vi "Update Table Data.vi"(8 "error in (no error)":errorcluster, 9 "Stream Names":string[](array[string]), 10 "Data":waveform(dbl)[](array[waveform]), 11 "Plugin in":refnum<class "Historical Table.lvclass">) -> (0 "error out":errorcluster, 3 "Plugin out":refnum<class "Historical Table.lvclass">)   [LabVIEW 2024, in "Historical Table.lvlib" / "Historical Table.lvclass"]
uses:
  Historical Table.lvclass
  Historical Table.lvclass/Historical Table.ctl
  <vilib>/FlexLogger/SDK/PluginSDK.lvlibp
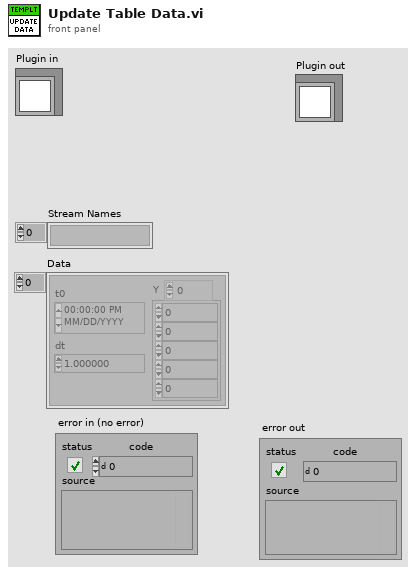
[diagram p1: front panel]
types:
  T1 = enum32{"Invalid", "Standard", "Closed", "Hidden", "Minimized", "Maximized"}
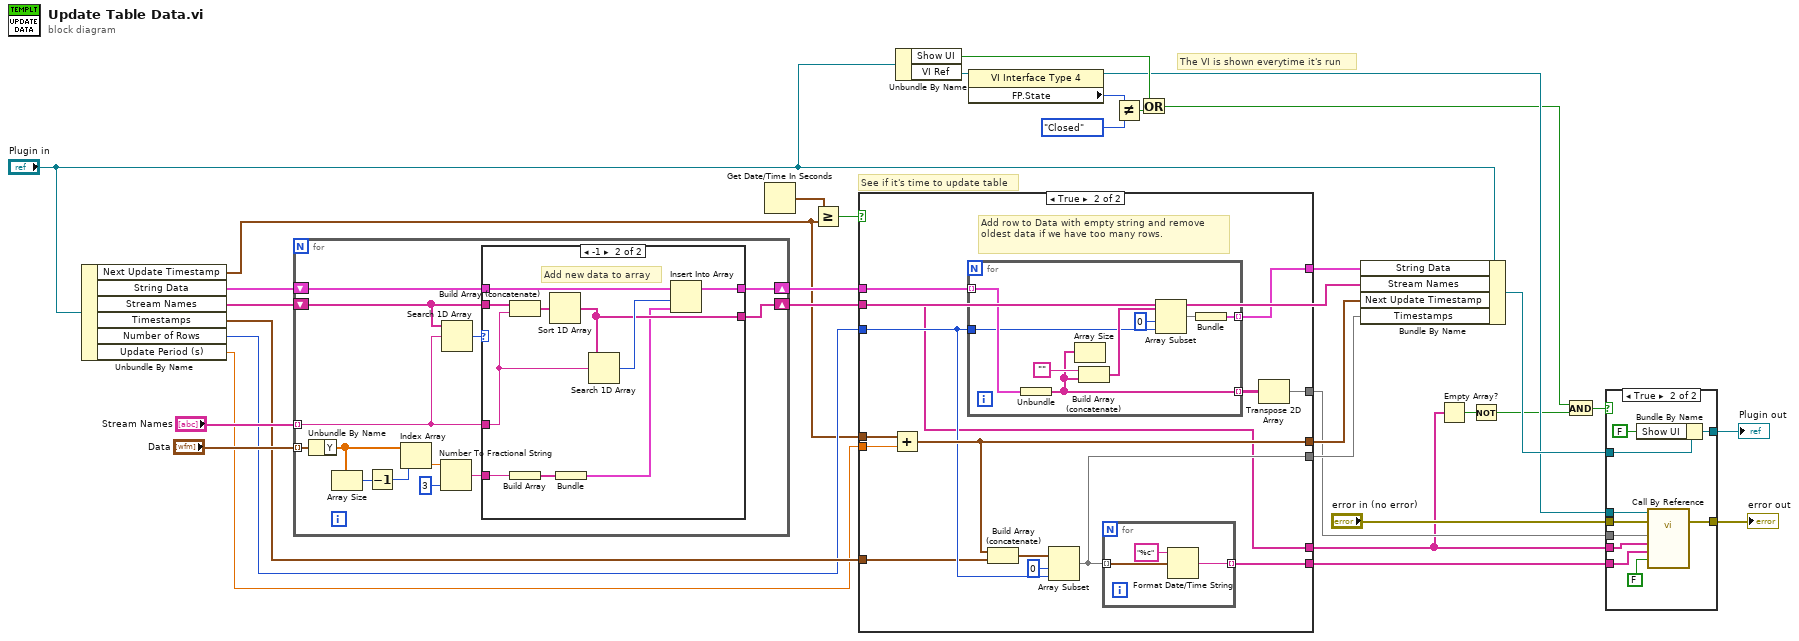
[diagram p0: block diagram]
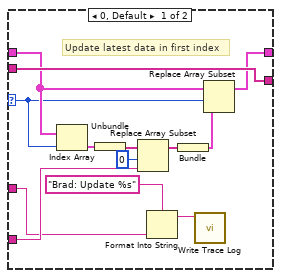
[diagram p3: hidden frame]
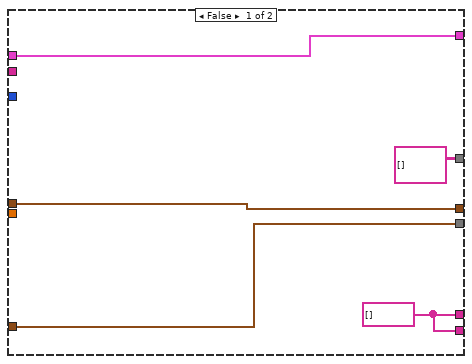
[diagram p4: hidden frame]
diagram:
  # "The VI is shown everytime it's run"
  # "See if it's time to update table"
  n1 = Unbundle By Name("Plugin in") -> ("Next Update Timestamp"=w4:timestamp, "String Data"=w31:cluster{"Data":string[]}[], "Stream Names"=w30:string[], "Timestamps"=w28:timestamp[], "Number of Rows"=w26:i32, "Update Period (s)"=w25:dbl)
  n2 = for {
    tunnel: "Data" -> [w41] mode=indexing
    tunnel: "Stream Names" -> [w45] mode=indexing
    shift-right: [w35] -> w29
    shift-left: w31 -> [w37]
    shift-right: [w34] -> w24
    shift-left: w30 -> [w36]
    n3 = Unbundle By Name(w41) -> ("Y"=w39:dbl[])
    n4 = Array Size(array=w39) -> (size(s)=w38:i32)
    n5 = Decrement(x=w38) -> (x-1=w43:i32)
    n6 = Index Array(array=w39, index=w43) -> (element=w44:dbl)
    n7 = Number To Fractional String(number=w44, precision (6)=i16 3) -> (F-format string=w40:string)  [unwired: 2 in]
    n8 = Search 1D Array(1D array=w36, element=w45) -> (index of element=w46:i32)  [unwired: 1 in]
    n9 = case shown="-1" w46 {
      selector: w46 -> [w56 _]
      tunnel: w36 -> [w59 w69]
      tunnel: w45 -> [w47 w60]
      tunnel: w37 -> [w57 w67]
      tunnel: [w59 w65] -> w34
      tunnel: [w58 w64] -> w35
      tunnel: w40 -> [w53 w63]
      frame 0, Default {
        # "Update latest data in first index"
        n10 = Index Array(array=w57, index=w56) -> (element=w55:cluster{"Data":string[]})
        n11 = Unbundle(w55) -> ("Data"=w54:string[])
        n12 = Replace Array Subset(array=w54, new element=w53, index=0) -> (w51:string[])
        n13 = Format Into String(format string="Brad: Update %s", w47) -> (resulting string=w49:string)  [unwired: 2 in, 1 out]
        n14 = Bundle("Data"=w51) -> (w50:cluster{"Data":string[]})  [unwired: 1 in]
        n15 = call <vilib>:"Write Trace Log.vi"("Message"=w49) -> ()  [unwired: 10 in, 1 out]
        n16 = Replace Array Subset(array=w57, new element=w50, index=w56) -> (w58:cluster{"Data":string[]}[])
      }
      frame -1 {
        # "Add new data to array"
        n17 = Build Array (concatenate)(w69, w60) -> (w68:string[])
        n18 = Build Array(w63) -> (w62:string[])
        n19 = Sort 1D Array(array=w68) -> (sorted array=w65:string[])
        n20 = Bundle(w62) -> (w61:cluster{string[]})  [unwired: 1 in]
        n21 = Search 1D Array(1D array=w65, element=w60) -> (index of element=w66:i32)  [unwired: 1 in]
        n22 = Insert Into Array(array=w67, index=w66, new element=w61) -> (w64:cluster{"Data":string[]}[])
      }
    }
  }
  n23 = Get Date/Time In Seconds() -> (seconds since 1Jan1904=w5:timestamp)
  n24 = Greater Or Equal?(x=w5, y=w4) -> (x >= y?=w6:bool)
  n25 = case shown="True" w6 {
    tunnel: w4 -> [w74 w87]
    tunnel: [w74 w84] -> w23
    tunnel: w25 -> [_ w88]
    tunnel: w26 -> [_ w83]
    tunnel: w29 -> [w73 w81]
    tunnel: w28 -> [w72 w80]
    tunnel: [w73 w79] -> w27
    tunnel: w24 -> [_ w77]
    tunnel: [w72 w78] -> w22
    tunnel: [w71 w77] -> w3
    tunnel: [w71 w76] -> w15
    tunnel: [string[][] [] w75] -> w9
    frame False {
      w71 = string[] [] ("Stream Names")
    }
    frame True {
      # "Add row to Data with empty string and remove oldest data if we have too many rows."
      n26 = Add(x=w87, y=w88) -> (x+y=w84:timestamp)
      n27 = for {
        tunnel: w81 -> [w99] mode=indexing
        tunnel: w83 -> [w93]
        tunnel: [w92] -> w82 mode=indexing
        tunnel: [w94] -> w79 mode=indexing
        n28 = Unbundle(w99) -> ("Data"=w92:string[])
        n29 = Array Size(array=w92) -> ()  [unwired: 1 out]
        n30 = Build Array (concatenate)("", w92) -> (w97:string[])
        n31 = Array Subset(array=w97, index=0, length=w93) -> (w95:string[])
        n32 = Bundle(w95) -> (w94:cluster{string[]})  [unwired: 1 in]
      }
      n33 = Build Array (concatenate)(w84, w80) -> (w86:timestamp[])
      n34 = Array Subset(array=w86, index=0, length=w83) -> (w78:timestamp[])
      n35 = for {
        tunnel: w78 -> [w90] mode=indexing
        tunnel: [w89] -> w76 mode=indexing
        n36 = Format Date/Time String(time format string (%c)="%c", seconds (now)=w90) -> (date/time string=w89:string)  [unwired: 1 in]
      }
      n37 = Transpose 2D Array(2D array=w82) -> (transposed array=w75:string[][])
    }
  }
  n38 = Unbundle By Name("Plugin in") -> ("Show UI"=w18:bool, "VI Ref"=w19:refnum<vi>)
  n39 = property class="VI Interface Type 4"(reference=w19) -> (reference out=w11:refnum<vi>, "FP.State"=w21:T1)  [unwired: 1 in, 1 out]
  n40 = Not Equal?(x=w21, y=T1."Closed" ("Front Panel Window:State")) -> (x != y?=w17:bool)
  n41 = Or(x=w18, y=w17) -> (x .or. y?=w10:bool)
  n42 = Bundle By Name(cluster="Plugin in", "String Data"=w27, "Stream Names"=w24, "Next Update Timestamp"=w23, "Timestamps"=w22) -> (w14:refnum<class "Historical Table.lvclass">)
  n43 = Empty Array?(array=w3) -> (empty?=w8:bool)
  n44 = Not(x=w8) -> (.not. x?=w7:bool)
  n45 = And(x=w10, y=w7) -> (x .and. y?=w1:bool)
  n46 = case shown="True" w1 {
    tunnel: w9 -> [_ w111]
    tunnel: w3 -> [_ w110]
    tunnel: w15 -> [_ w109]
    tunnel: "error in (no error)" -> [w101 w107]
    tunnel: [w101 w106] -> w2
    tunnel: [w100 w104] -> w13
    tunnel: w14 -> [w100 w103]
    tunnel: w11 -> [_ w102]
    frame False {
    }
    frame True {
      n47 = Bundle By Name(cluster=w103, "Show UI"=FALSE) -> (w104:refnum<class "Historical Table.lvclass">)
      n48 = call-by-ref "?"(reference=w102, error in=w107, "Reset Table Data"=FALSE, "Row Headers"=w109, "Column Headers"=w110, "Table Data"=w111) -> (error out=w106:errorcluster)  [unwired: 8 in, 1 out]
    }
  }
  "Plugin out" <- w13
  "error out" <- w2
